vi "AttrGetFirmwareRev.vi"(5 "LogSuspend":bool, 8 "error in":errorcluster, 11 "UdsHandleIn":T1={"LogPath"=path "", "LogEnabled"=FALSE, "isOpen"=FALSE, "LogContent"="", "Adapter"="CAN0", "MCanHandle"={"MCanAdapter"=refnum}, "TransmittId"=0, "ReceiveId"=0}) -> (0 "error out":errorcluster, 2 "Value":string, 3 "UdsHandleOut":T1={"LogPath"=path "", "LogEnabled"=FALSE, "isOpen"=FALSE, "LogContent"="", "Adapter"="CAN0", "MCanHandle"={"MCanAdapter"=refnum}, "TransmittId"=0, "ReceiveId"=0})   [LabVIEW 2011, in "Konvolucio MUDS150628.lvlib"]
uses:
  <instrlib>/Konvolucio MUDS150628/Konvolucio MUDS150628.lvlib
  <instrlib>/Konvolucio MUDS150628/Types/UdsHandleType.ctl
  <instrlib>/Konvolucio MCAN120803/Types/MCanHandleType.ctl
  C:/Program Files/National Instruments/LabVIEW 2011/instr.lib/Konvolucio MCAN120803/Private/Konvolucio.MCAN120803.dll
  Konvolucio MCAN120803/Private/Konvolucio.MCAN120803.dll
  <instrlib>/Konvolucio MCAN120803/Konvolucio MCAN120803.lvlib
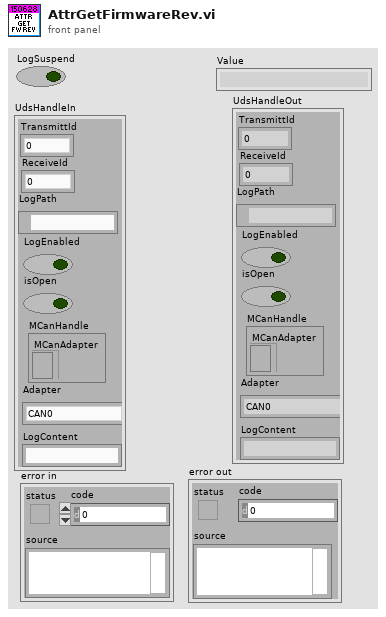
[diagram p1: front panel]
types:
  T1 = typedef "Konvolucio MUDS150628.lvlib/UdsHandleType.ctl" = cluster{"LogPath":path, "LogEnabled":bool, "isOpen":bool, "LogContent":string, "Adapter":string, "MCanHandle":T2, "TransmittId":u32, "ReceiveId":u32}
  T2 = typedef "Konvolucio MCAN120803.lvlib/MCanHandleType.ctl" = cluster{"MCanAdapter":refnum<k24>}
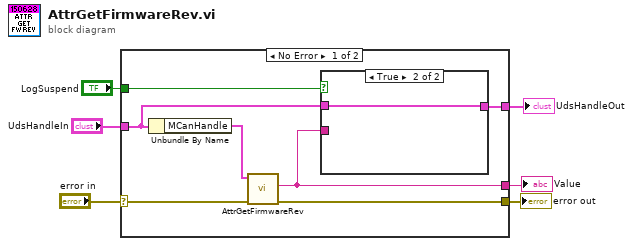
[diagram p0: block diagram]
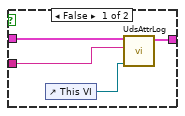
[diagram p2: hidden frame]
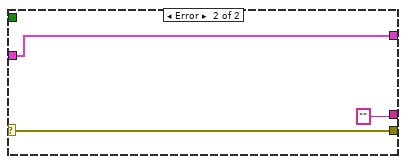
[diagram p3: hidden frame]
diagram:
  n1 = case shown="No Error" "error in" {
    selector: "error in" -> [w10 w21]
    tunnel: [w9 w21] -> w6
    tunnel: "UdsHandleIn" -> [w13 w20]
    tunnel: [w12 w20] -> w3
    tunnel: "LogSuspend" -> [w11 _]
    tunnel: [w7 "" ("Attributes.FirmwareRev")] -> w1
    frame No Error {
      n2 = Unbundle By Name(w13) -> ("MCanHandle"=w8:T2)
      n3 = call <instrlib>:"AttrGetFirmwareRev.vi"("error in"=w10, "MCanHandleIn"=w8) -> ("error out"=w9:errorcluster, "Value"=w7:string)  [unwired: 7 in, 1 out]
      n4 = case shown="True" w11 {
        tunnel: w13 -> [w17 w18]
        tunnel: [w16 w18] -> w12
        tunnel: w7 -> [w14 _]
        frame False {
          n5 = control-ref of="This VI"() -> (w15:refnum<vi>)
          n6 = call <instrlib>:"UdsAttrLog.vi"("This VI"=w15, "Content"=w14, "UdsHandleIn"=w17) -> ("UdsHandleOut"=w16:T1)  [unwired: 8 in]
        }
        frame True {
        }
      }
    }
    frame Error {
    }
  }
  "Value" <- w1
  "error out" <- w6
  "UdsHandleOut" <- w3
